vi "SET_LEVEL_KEITHLEY2470.vi"(8 "error in (no error)":errorcluster, 10 "Cluster":T1={"VISA resource name"="", "Function (0: Volts) 1"=1, "Function (0: Volts) 2 "=0, "Enable Auto Range (T:Enable)"=TRUE, "Source Mode  (0: Voltage)"=0, "Source Level (0)"=0.0, "Source Limit Level (0.1)"=0.01} {"Source Limit Level (0.1)" format="%#_13g"; "Source Level (0)" format="%#_13g"; "Source Mode  (0: Voltage)" items=["Voltage", "Current"]; "Function (0: Volts) 2" items=["Volts", "Current", "Resistance"]; "Function (0: Volts) 1" items=["Volts", "Current", "Resistance"]}, 11 "VISA resource name":refnum<visa-resource-name>) -> (0 "error out":errorcluster, 3 "VISA resource name out":refnum<visa-resource-name>)   [LabVIEW 2019]
uses:
  Type Definition/handle_Para.ctl
  <instrlib>/Keithley 2450/Keithley 2450.lvlib
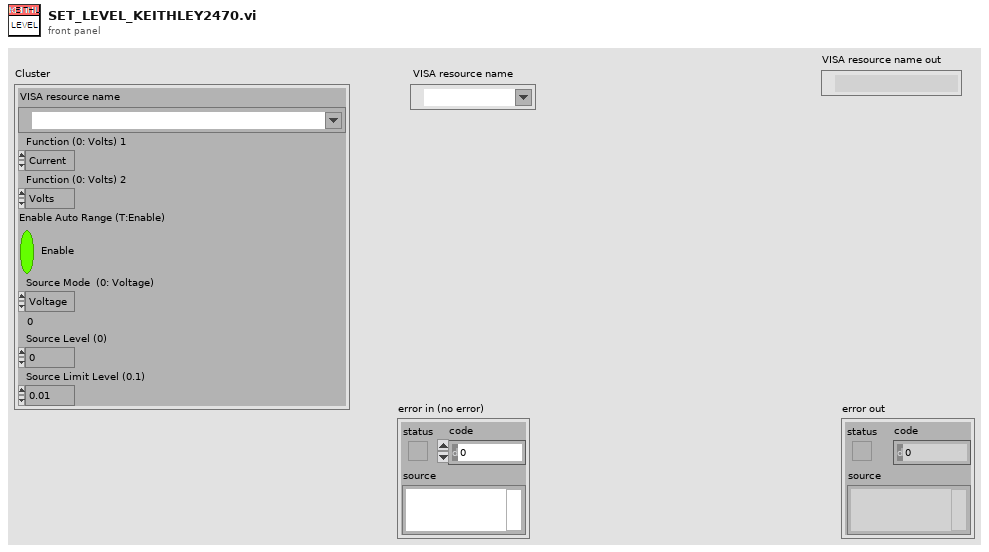
[diagram p1: front panel]
types:
  T1 = typedef "handle_Para.ctl" = cluster{"VISA resource name":refnum<visa-resource-name>, "Function (0: Volts) 1":u16, "Function (0: Volts) 2 ":u16, "Enable Auto Range (T:Enable)":bool, "Source Mode  (0: Voltage)":u16, "Source Level (0)":dbl, "Source Limit Level (0.1)":dbl}
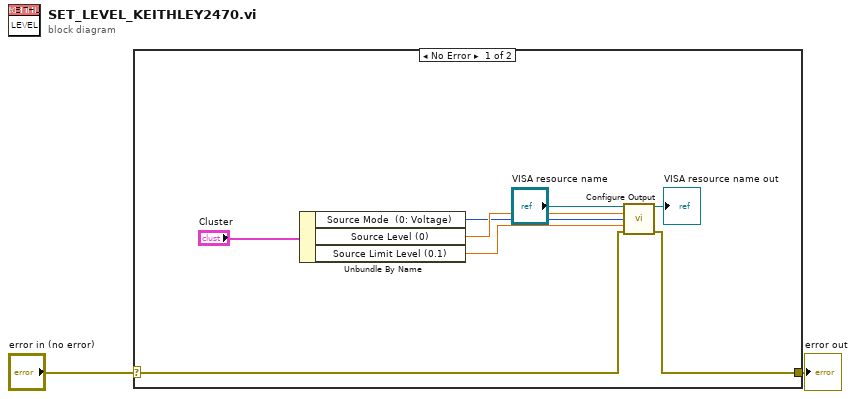
[diagram p0: block diagram]
diagram:
  n1 = case shown="No Error" "error in (no error)" {
    selector: "error in (no error)" -> [w6 w11]
    tunnel: [w5 w11] -> w1
    frame No Error {
      n2 = Unbundle By Name("Cluster") -> ("Source Mode  (0: Voltage)"=w8:u16, "Source Level (0)"=w9:dbl, "Source Limit Level (0.1)"=w10:dbl)
      n3 = call <instrlib>:"Configure Output.vi"("VISA resource name"="VISA resource name", "Source Level (0)"=w9, "Source Mode  (0: Voltage)"=w8, "Source Limit Level (0.1)"=w10, "error in (no error)"=w6) -> ("VISA resource name out"=→"VISA resource name out":refnum<visa-resource-name>, "error out"=w5:errorcluster)  [unwired: 9 in]
    }
    frame Error {
    }
  }
  "error out" <- w1
